vi "ep_Read Status Channel Info.vi"(8 "error in (no error)":errorcluster, 11 "task in":T2={"file refnums"=[], "Data Object"=refnum, "config info"={"station_name"="", "rec_dev_id"="", "rev_year"=1999.0, "TT"=0, "##A"=0, "##D"=0, "analog channel info"=[], "status channel info"=[], "lf"=50.0, "nrates"=0, "samp info"=[], "initial timestamp"=timestamp(0 s since 1904-01-01), "trigger timestamp"=timestamp(0 s since 1904-01-01), "ft"=enum."Binary", "timemult"=1.0}, "public inf content"={"Source"="", "Record Type"=enum."Unknown", "Phase ID"="", "Event Description"="", "Device ID"="", "Distance of Fault"=-1.0, "Distance Unit"=enum."Miles", "Max_Current"=inf, "Min_Current"=-inf, "Max_Voltage"=inf, "Min_Voltage"=-inf, "EventNoteCount"=0, "Event Information"=[]}, "private inf content"=[], "internal buffers"={"start index"=1, "config to public inf"=enum."disabled", "static config info"="", "static file_des record inf"="", "static file_des channel inf"="", "public inf"="", "private inf"=""}} {"public inf content"."Event Information"."min sample number" max=9999999999; "public inf content"."Event Information"."max sample number" max=9999999999; "config info"."nrates" max=999; "config info"."status channel info"."Dn" min=1 max=999999; "config info"."analog channel info"."An" min=1 max=999999; "config info"."trigger timestamp" format="%<%H:%M:%S%6u\n%d/%m/%Y>T"; "config info"."initial timestamp" format="%<%H:%M:%S%6u\n%d/%m/%Y>T"; "config info"."##D" max=999999; "config info"."##A" max=999999; "config info"."TT" min=1 max=999999; "config info"."rev_year" min=1999.0 max=1999.0}) -> (0 "error out":errorcluster, 2 "status channel info":T1[](array[typedef]), 3 "task out":T2={"file refnums"=[], "Data Object"=refnum, "config info"={"station_name"="", "rec_dev_id"="", "rev_year"=1999.0, "TT"=0, "##A"=0, "##D"=0, "analog channel info"=[], "status channel info"=[], "lf"=50.0, "nrates"=0, "samp info"=[], "initial timestamp"=timestamp(0 s since 1904-01-01), "trigger timestamp"=timestamp(0 s since 1904-01-01), "ft"=enum."Binary", "timemult"=1.0}, "public inf content"={"Source"="", "Record Type"=enum."Unknown", "Phase ID"="", "Event Description"="", "Device ID"="", "Distance of Fault"=-1.0, "Distance Unit"=enum."Miles", "Max_Current"=inf, "Min_Current"=-inf, "Max_Voltage"=inf, "Min_Voltage"=-inf, "EventNoteCount"=0, "Event Information"=[]}, "private inf content"=[], "internal buffers"={"start index"=1, "config to public inf"=enum."disabled", "static config info"="", "static file_des record inf"="", "static file_des channel inf"="", "public inf"="", "private inf"=""}} {"public inf content"."Event Information"."min sample number" max=9999999999; "public inf content"."Event Information"."max sample number" max=9999999999; "config info"."nrates" max=999; "config info"."status channel info"."Dn" min=1 max=999999; "config info"."analog channel info"."An" min=1 max=999999; "config info"."trigger timestamp" format="%<%H:%M:%S%6u\n%d/%m/%Y>T"; "config info"."initial timestamp" format="%<%H:%M:%S%6u\n%d/%m/%Y>T"; "config info"."##D" max=999999; "config info"."##A" max=999999; "config info"."TT" min=1 max=999999; "config info"."rev_year" min=1999.0 max=1999.0})   [LabVIEW 2014, in "NI_EP_COMTRADE.lvlib"]
uses:
  <vilib>/addons/Electrical Power/File IO/NI_EP_COMTRADE.lvlib
  <vilib>/addons/Electrical Power/File IO/COMTRADE/typedefs/ep_Task.ctl
  <vilib>/addons/Electrical Power/File IO/COMTRADE/typedefs/ep_Config Info.ctl
  <vilib>/addons/Electrical Power/File IO/COMTRADE/typedefs/ep_Analog Channel Info.ctl
  <vilib>/addons/Electrical Power/File IO/COMTRADE/typedefs/ep_Status Channel Info.ctl
  <vilib>/addons/Electrical Power/File IO/COMTRADE/typedefs/ep_File Format.ctl
  <vilib>/addons/Electrical Power/File IO/COMTRADE/typedefs/ep_Public Inf Content.ctl
  <vilib>/addons/Electrical Power/File IO/COMTRADE/typedefs/ep_Public Event Inf.ctl
  <vilib>/addons/Electrical Power/File IO/COMTRADE/typedefs/ep_Private Inf Content.ctl
  <vilib>/addons/Electrical Power/File IO/COMTRADE/typedefs/ep_Status Channel Info (UI).ctl
  <vilib>/Platform/storage/Storage.llb/Get Property (Storage Refnums).vi
  <vilib>/Platform/storage/Storage.llb/Get Property (I32).vi
  <vilib>/Platform/storage/Storage.llb/Get Property (String).vi
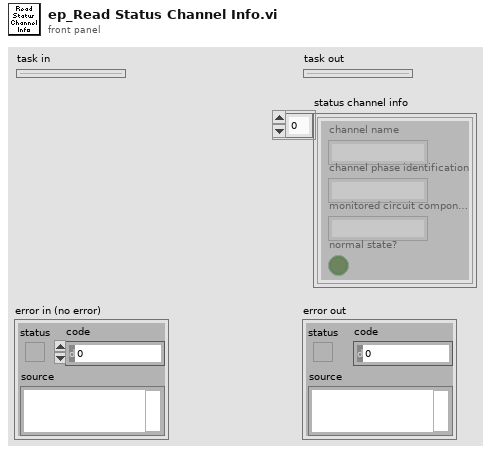
[diagram p1: front panel]
types:
  T1 = typedef "NI_EP_COMTRADE.lvlib/ep_Status Channel Info (UI).ctl" = cluster{"channel name":string, "channel phase identification":string, "monitored circuit component":string, "normal state?":bool}
  T2 = typedef "NI_EP_COMTRADE.lvlib/ep_Task.ctl" = cluster{"file refnums":refnum<file>[], "Data Object":refnum<k20>, "config info":T3, "public inf content":T7, "private inf content":T9, "internal buffers":cluster{"start index":u32, "config to public inf":enum16{"disabled", "enabled", "buffered"}, "static config info":string, "static file_des record inf":string, "static file_des channel inf":string, "public inf":string, "private inf":string}}
  T3 = typedef "NI_EP_COMTRADE.lvlib/ep_Config Info.ctl" = cluster{"station_name":string, "rec_dev_id":string, "rev_year":dbl, "TT":u32, "##A":u32, "##D":u32, "analog channel info":T4[], "status channel info":T5[], "lf":sgl, "nrates":u16, "samp info":cluster{"samp":sgl, "endsamp":u32}[], "initial timestamp":timestamp, "trigger timestamp":timestamp, "ft":T6, "timemult":sgl}
  T4 = typedef "NI_EP_COMTRADE.lvlib/ep_Analog Channel Info.ctl" = cluster{"An":u32, "ch_id":string, "ph":string, "ccbm":string, "uu":string, "a":sgl, "b":sgl, "skew":sgl, "min":i32, "max":i32, "primary":sgl, "secondary":sgl, "PS":enum16{"P", "S"}}
  T5 = typedef "NI_EP_COMTRADE.lvlib/ep_Status Channel Info.ctl" = cluster{"Dn":u32, "ch_id":string, "ph":string, "ccbm":string, "Y":bool}
  T6 = typedef "NI_EP_COMTRADE.lvlib/ep_File Format.ctl" = enum16{"ASCII", "Binary"}
  T7 = typedef "NI_EP_COMTRADE.lvlib/ep_Public Inf Content.ctl" = cluster{"Source":string, "Record Type":enum16{"Fault", "Unknown", "Misoperation", "Close", "Trip", "Reclose", "Power swing", "Simulation"}, "Phase ID":string, "Event Description":string, "Device ID":string, "Distance of Fault":dbl, "Distance Unit":enum16{"Miles", "Kilometers", "Percent of line", "Percent of setting", "Ohms"}, "Max_Current":dbl, "Min_Current":dbl, "Max_Voltage":dbl, "Min_Voltage":dbl, "EventNoteCount":u32, "Event Information":T8[]}
  T8 = typedef "NI_EP_COMTRADE.lvlib/ep_Public Event Inf.ctl" = cluster{"channel number":u32, "max value":dbl, "min value":dbl, "max sample number":u64, "min sample number":u64, "max sample text":string[], "min sample text":string[]}
  T9 = typedef "NI_EP_COMTRADE.lvlib/ep_Private Inf Content.ctl" = cluster{"Section Header":string, "Entry Names":string[], "Entry Values":string[]}[]
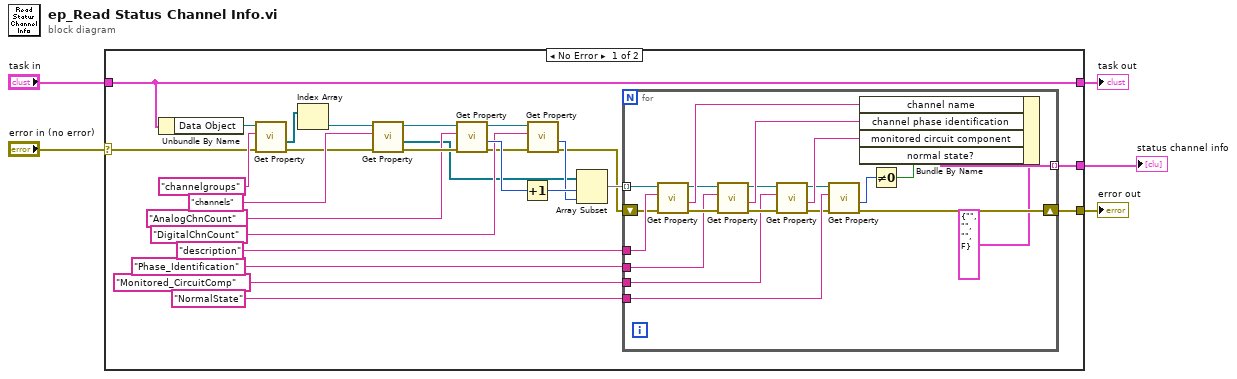
[diagram p0: block diagram]
diagram:
  n1 = case shown="No Error" "error in (no error)" {
    selector: "error in (no error)" -> [w27 w53]
    tunnel: [w10 w53] -> w4
    tunnel: [w31 w52] -> w3
    tunnel: "task in" -> [w31 w52]
    tunnel: [w9 _] -> w1
    frame No Error {
      n2 = Unbundle By Name(w31) -> ("Data Object"=w30:refnum<k20>)
      n3 = call-poly <vilib>:"Get Property.vi"("error in (no error)"=w27, "Property name"="channelgroups", "storage refnum"=w30) -> ("error out"=w6:errorcluster, "Value"=w28:refnum<k20>[])  [unwired: 6 in, 1 out]
      n4 = Index Array(array=w28) -> (element=w26:refnum<k20>)  [unwired: 1 in]
      n5 = call-poly <vilib>:"Get Property.vi"("error in (no error)"=w6, "Property name"="channels", "storage refnum"=w26) -> ("error out"=w23:errorcluster, "Value"=w16:refnum<k20>[], "storage refnum out"=w24:refnum<k20>)  [unwired: 6 in]
      n6 = call-poly <vilib>:"Get Property.vi"("error in (no error)"=w23, "Property name"="AnalogChnCount", "storage refnum"=w24) -> ("error out"=w8:errorcluster, "Value"=w20:i32, "storage refnum out"=w19:refnum<k20>)  [unwired: 6 in]
      n7 = Increment(x=w20) -> (x+1=w21:i32)
      n8 = call-poly <vilib>:"Get Property.vi"("error in (no error)"=w8, "Property name"="DigitalChnCount", "storage refnum"=w19) -> ("error out"=w7:errorcluster, "Value"=w17:i32)  [unwired: 6 in, 1 out]
      n9 = Array Subset(array=w16, index=w21, length=w17) -> (w15:refnum<k20>[])
      n10 = for {
        tunnel: w15 -> [w51] mode=indexing
        tunnel: "description" ("Property name") -> [w50]
        tunnel: "Phase_Identification" ("Property name") -> [w48]
        tunnel: "Monitored_CircuitComp" ("Property name") -> [w34]
        tunnel: "NormalState" ("Property name") -> [w47]
        shift-right: [w41] -> w10
        shift-left: w7 -> [w46]
        tunnel: [w40] -> w9 mode=indexing
        n11 = call-poly <vilib>:"Get Property.vi"("error in (no error)"=w46, "Property name"=w50, "storage refnum"=w51) -> ("error out"=w49:errorcluster, "Value"=w45:string, "storage refnum out"=w39:refnum<k20>)  [unwired: 6 in]
        n12 = call-poly <vilib>:"Get Property.vi"("error in (no error)"=w49, "Property name"=w48, "storage refnum"=w39) -> ("error out"=w35:errorcluster, "Value"=w44:string, "storage refnum out"=w36:refnum<k20>)  [unwired: 6 in]
        n13 = call-poly <vilib>:"Get Property.vi"("error in (no error)"=w35, "Property name"=w34, "storage refnum"=w36) -> ("error out"=w33:errorcluster, "Value"=w38:string, "storage refnum out"=w37:refnum<k20>)  [unwired: 6 in]
        n14 = call-poly <vilib>:"Get Property.vi"("error in (no error)"=w33, "Property name"=w47, "storage refnum"=w37) -> ("error out"=w41:errorcluster, "Value"=w43:i32)  [unwired: 6 in, 1 out]
        n15 = Not Equal To 0?(x=w43) -> (x != 0?=w42:bool)
        n16 = Bundle By Name(cluster=T1 {"channel name"="", "channel phase identification"="", "monitored circuit component"="", "normal state?"=FALSE}, "channel name"=w45, "channel phase identification"=w44, "monitored circuit component"=w38, "normal state?"=w42) -> (w40:T1)
      }
    }
    frame Error {
    }
  }
  "error out" <- w4
  "task out" <- w3
  "status channel info" <- w1
